vi "適應性控制_輸入權重係數+數位積分_隔振V2(實際控制).vi"() -> ()   [LabVIEW 2010]
uses:
  <vilib>/DAQmx/read.llb/DAQmx Read (Analog DBL 1Chan 1Samp).vi
  <vilib>/DAQmx/write.llb/DAQmx Write (Analog DBL 1Chan 1Samp).vi
  <vilib>/DAQmx/create/channels.llb/DAQmx Create Channel (AI-Voltage-Basic).vi
  <vilib>/DAQmx/configure/timing.llb/DAQmx Timing (Sample Clock).vi
  <vilib>/DAQmx/create/channels.llb/DAQmx Create Channel (AO-Voltage-Basic).vi
  <vilib>/daqmx/miscellaneous.llb/DAQmx Fill In Error Info.vi
  <vilib>/measure/maspectr.llb/FFT Spectrum (Mag-Phase) for 1 Chan.vi
  <vilib>/measure/NI_MAPro.lvlib
panel:
  in  "權重":dbl[][](array[numeric])=array3077x82[252314 elements]
  in  "輸出DC濾除":dbl
  out "當前權重":dbl[](array[numeric])
  in  "相位":dbl
  in  "頻率":dbl
  in  "averaging parameters":T1={"averaging mode"=enum."No averaging", "weighting mode"=enum."Exponential", "number of averages"=10} {"number of averages" min=1}
  in  "I增益":dbl
  out "magnitude":cluster{"f0":dbl, "df":dbl, "magnitude":dbl[]} {"magnitude" format="%.2p"; "f0" format="%0.2p"; "df" format="%0.2p"}
  out "Waveform Graph":cluster{"f0":dbl, "df":dbl, "magnitude":dbl[]}(graph)
  in  "DAQ input":tag
  in  "DAQ output":tag
  in  "平均數":i32=1
  in  "ÂoDC«á©ñ¤j":dbl=1.0
  in  "Kp":dbl
  out "當下誤差":dbl=0.1 format="%#_13g"
  out "模擬輸入x(t)":dbl[][](graph)
  out "理想與FIR輸出":dbl[][](graph)
  out "message":string=" INSTRUCTIONS:\r\rNormal Use:  When using subVIs that incorporate the error in/error out (or error I/O) structure, place this handler where you want to inform the user of an error, typically at the end of the I/O data path, as the last action of the program.  If the error in error? is ERROR, the handler creates a message describing the error and its source.  If the type of dialog = 1 (default), the message is displayed to the user, who can only acknowedge it.  If the type = 2, the user can acknowledge the message or abort execution; aborting a program with active I/O is not recommended.  If the type = 0, no message is displayed; this is used to process the error programmatically, and the error out cluster elements are wired to individual terminals for that reason.  \r\rOther Use:\n\r\nlocal testing.  To test the error code of a subVI or function that does not have the error I/O structure, you can wire its error code and a source string to the local error code and error source inputs.  If error in error? indicates no error and error code is not equal to 0, the local code and source are substituted for the error in values, and error? is set TRUE (ERROR)."
  out "誤差":dbl(graph)
  out "while平均運行時間":dbl
  out "收斂time":dbl
  out "各頻率誤差已達標準":bool
  in  "各頻率誤差低於多少亮燈":dbl=0.1 format="%#_13g"
  in  "order":i32=80
  in  "取樣頻率":dbl=1000.0 min=1.0 max=1000.0 step=1.0
  in  "stop":bool
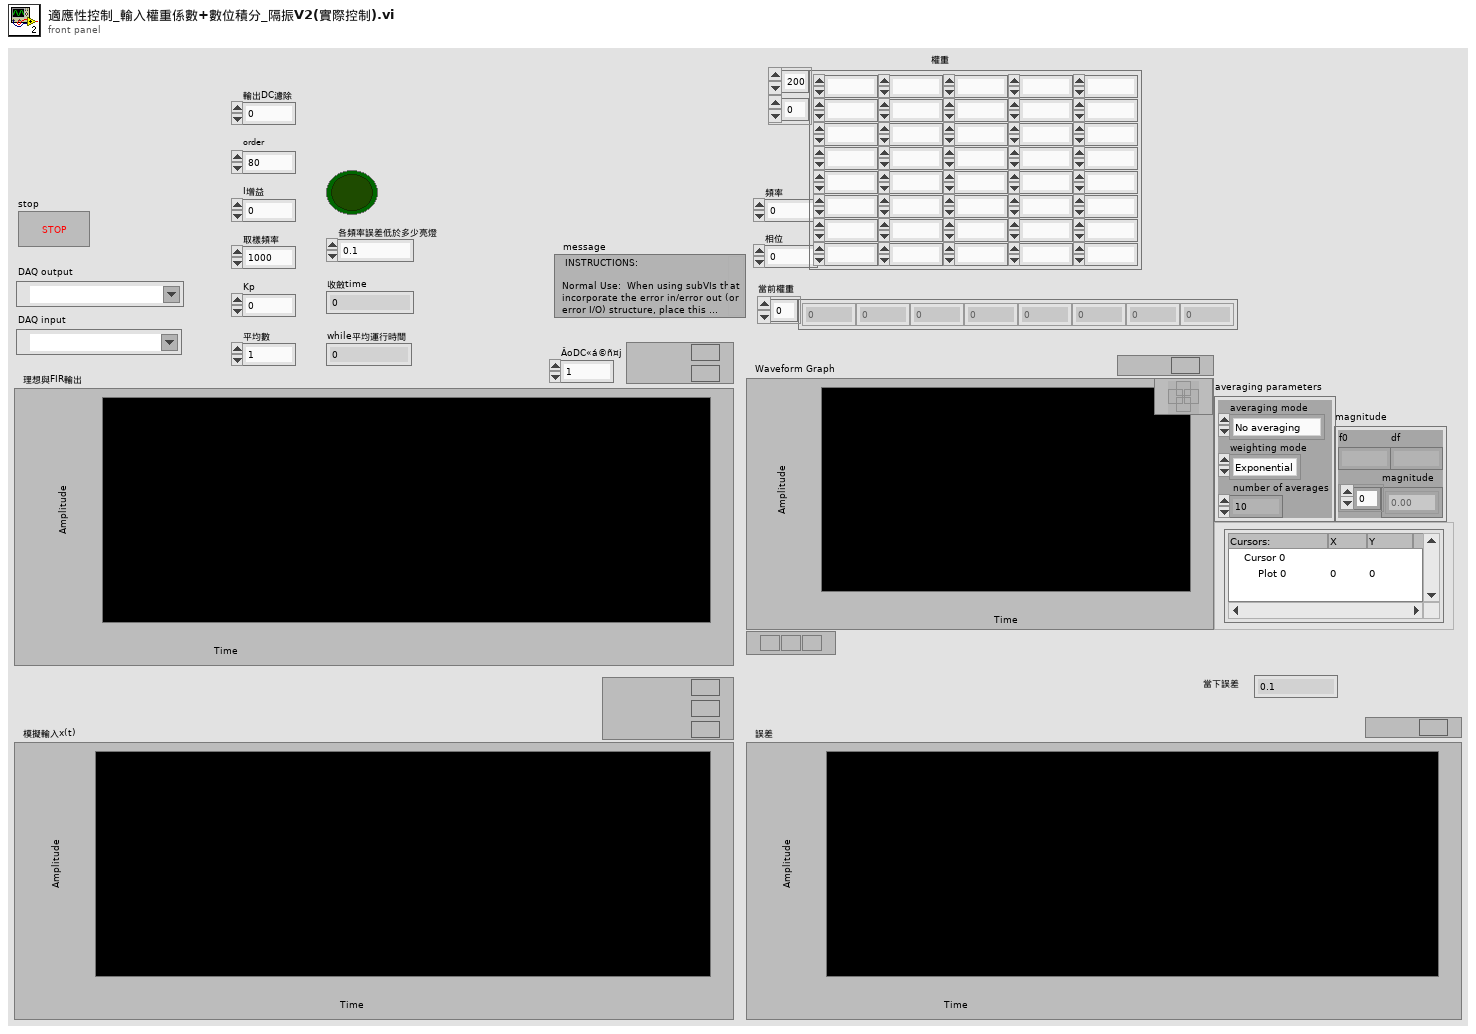
[diagram p1: front panel]
types:
  T1 = cluster{"averaging mode":enum16{"No averaging", "Vector averaging", "RMS averaging", "Peak hold"}, "weighting mode":enum16{"Linear", "Exponential"}, "number of averages":u32}
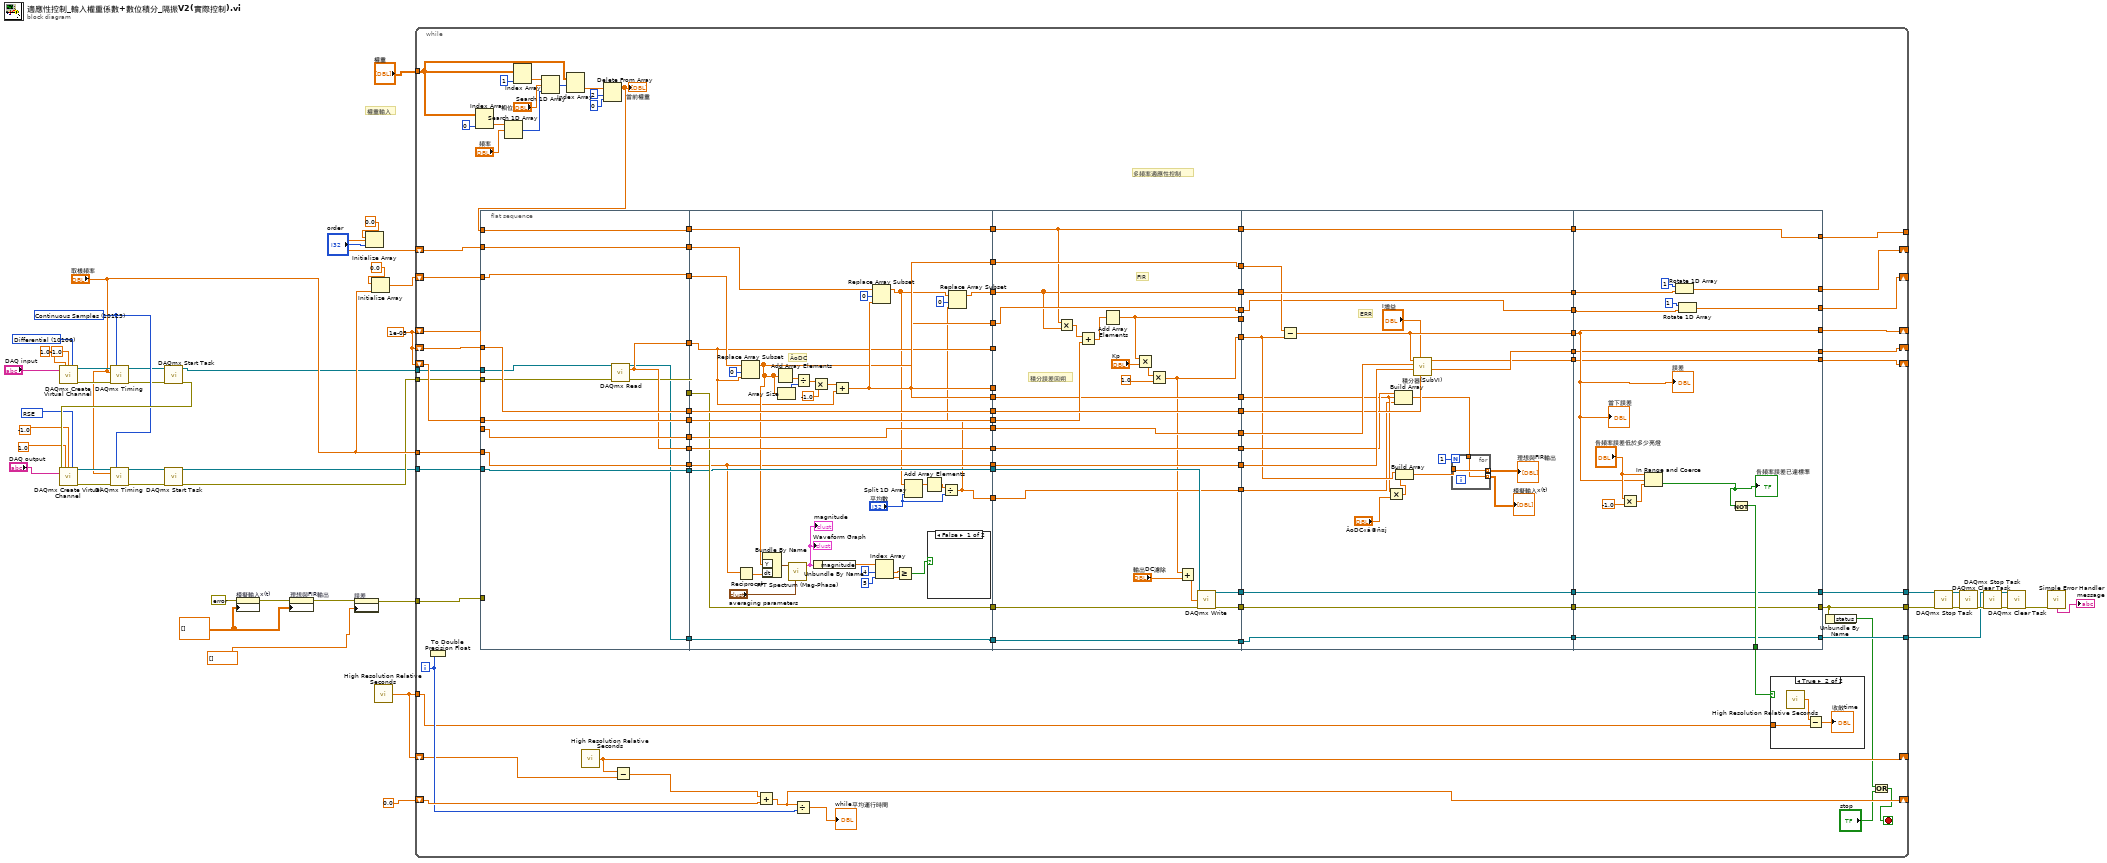
[diagram p0: block diagram]
diagram:
  w29 = 10123 items=["Finite Samples"=10178, "Continuous Samples"=10123, "Hardware Timed Single Point"=12522] ("sample mode")
  w26 = 10083 items=["Default"=-1, "RSE"=10083, "Differential"=10106, "Pseudodifferential"=12529] ("output terminal configuration")
  w25 = 10106 items=["default"=-1, "RSE"=10083, "NRSE"=10078, "Differential"=10106, "Pseudodifferential"=12529] ("input terminal configuration")
  w37 = 1e-05 ("x")
  w33 = dbl[][] [] ("History Data")
  # "權重輸入"
  n1 = call-poly <vilib>:"DAQmx Create Virtual Channel.vi"("maximum value"=1.0, "minimum value"=-1.0, "input terminal configuration"=w25, "physical channels"="DAQ input") -> ("task out"=w17:refnum<k21>, "error out"=w20:errorcluster)  [unwired: 10 in]
  n2 = call-poly <vilib>:"DAQmx Timing.vi"("task/channels in"=w17, "sample mode"=w29, "rate"="取樣頻率", "error in"=w20) -> ("task out"=w18:refnum<k21>, "error out"=w19:errorcluster)  [unwired: 10 in]
  n3 = call <vilib>:"DAQmx Start Task.vi"("task/channels in"=w18, "error in"=w19) -> ("task out"=w15:refnum<k21>, "error out"=w32:errorcluster)  [unwired: 12 in]
  n4 = call-poly <vilib>:"DAQmx Create Virtual Channel.vi"("maximum value"=1.0, "minimum value"=-1.0, "output terminal configuration"=w26, "physical channels"="DAQ output", "error in"=w32) -> ("task out"=w24:refnum<k21>, "error out"=w21:errorcluster)  [unwired: 9 in]
  n5 = call-poly <vilib>:"DAQmx Timing.vi"("task/channels in"=w24, "sample mode"=w29, "rate"="取樣頻率", "error in"=w21) -> ("task out"=w23:refnum<k21>, "error out"=w22:errorcluster)  [unwired: 10 in]
  n6 = call <vilib>:"DAQmx Start Task.vi"("task/channels in"=w23, "error in"=w22) -> ("task out"=w13:refnum<k21>, "error out"=w14:errorcluster)  [unwired: 12 in]
  n7 = property on="模擬輸入x(t)" class="WFChart (strict)"(error in=errorcluster {"status"=FALSE, "code"=0, "source"=""} ("error constant"), "History Data"=w33) -> (error out=w41:errorcluster)  [unwired: 1 in, 1 out]
  n8 = property on="理想與FIR輸出" class="WFChart (strict)"(error in=w41, "History Data"=w33) -> (error out=w42:errorcluster)  [unwired: 1 in, 1 out]
  n9 = property on="誤差" class="WFChart (strict)"(error in=w42, "History Data"=dbl[] []) -> (error out=w44:errorcluster)  [unwired: 1 in, 1 out]
  n10 = Initialize Array(0.0 ("element"), "order") -> (w36:dbl[])
  n11 = Initialize Array(0.0 ("element"), "取樣頻率") -> (w34:dbl[])
  n12 = call <vilib>:"High Resolution Relative Seconds.vi"() -> ("relative seconds"=w46:dbl)
  n13 = while {
    shift-right: [w118] -> _
    shift-left: w36 -> [w142]
    tunnel: w46 -> [w126]
    shift-right: [w127] -> _
    shift-left: w46 -> [w125]
    shift-right: [w128] -> _
    shift-left: 0.0 -> [w130]
    tunnel: w44 -> [w122]
    shift-right: [w116] -> _
    shift-left: w37 -> [w112]
    shift-right: [w108] -> _
    shift-left: w37 -> [w103]
    shift-right: [w102] -> _
    shift-left: w37 -> [w98]
    tunnel: "取樣頻率" -> [w97]
    tunnel: [w92] -> _
    shift-right: [w89] -> _
    shift-left: w34 -> [w91]
    tunnel: w15 -> [w81]
    tunnel: w14 -> [w80]
    tunnel: w13 -> [w79]
    tunnel: [w74] -> w7
    tunnel: [w64] -> w6
    tunnel: [w67] -> w5
    tunnel: "權重" -> [w49]
    i -> [w129]
    stop <- w66 stop-if-true
    # "多頻率適應性控制"
    n14 = To Double Precision Float(number=w129) -> ()  [unwired: 1 out]
    n15 = Index Array(array=w49, index (col)=0 ("disabled index (col)")) -> (element=w59:dbl[])  [unwired: 1 in]
    n16 = flat-sequence {
      tunnel: [w159] -> w143
      tunnel: w142 -> [w159]
      tunnel: [w150] -> w141
      tunnel: [w158] -> w138
      tunnel: w48 -> [w158]
      tunnel: w122 -> [_]
      tunnel: [w150] -> w119
      tunnel: [w157] -> w113
      tunnel: w112 -> [w157]
      tunnel: [w156] -> w109
      tunnel: w97 -> [w156]
      tunnel: [w155] -> w104
      tunnel: w103 -> [w155]
      tunnel: [w154] -> w99
      tunnel: w98 -> [w154]
      tunnel: [w149] -> w96
      tunnel: w91 -> [w153]
      tunnel: [w153] -> w90
      tunnel: w81 -> [w152]
      tunnel: w80 -> [w151]
      tunnel: w79 -> [w148]
      tunnel: [w148] -> w77
      tunnel: [w147] -> w70
      tunnel: w143 -> [w196]
      tunnel: w141 -> [w164]
      tunnel: [w162] -> w140
      tunnel: [w197] -> w139
      tunnel: w138 -> [w197]
      tunnel: [w190] -> w123
      tunnel: [w195] -> w120
      tunnel: w119 -> [w195]
      tunnel: [w193] -> w114
      tunnel: w113 -> [w193]
      tunnel: [w167] -> w110
      tunnel: w109 -> [w167]
      tunnel: [w192] -> w105
      tunnel: w104 -> [w192]
      tunnel: [w191] -> w100
      tunnel: w99 -> [w191]
      tunnel: w96 -> [w190]
      tunnel: [w182] -> w94
      tunnel: w90 -> [w188]
      tunnel: [w169] -> w86
      tunnel: [w182] -> w85
      tunnel: [w182] -> w83
      tunnel: [w160] -> w82
      tunnel: [w178] -> w78
      tunnel: w77 -> [w178]
      tunnel: [w177] -> w71
      tunnel: w70 -> [w177]
      tunnel: [w164] -> w61
      tunnel: w140 -> [w202]
      tunnel: w139 -> [w204]
      tunnel: [w204] -> w137
      tunnel: [w203] -> w136
      tunnel: [w202] -> w135
      tunnel: w123 -> [w209]
      tunnel: [w201] -> w121
      tunnel: w120 -> [w201]
      tunnel: [w222] -> w115
      tunnel: w114 -> [w222]
      tunnel: [w221] -> w111
      tunnel: w110 -> [w221]
      tunnel: [w220] -> w106
      tunnel: w105 -> [w220]
      tunnel: w100 -> [w218]
      tunnel: [w214] -> w95
      tunnel: w94 -> [w214]
      tunnel: [w198] -> w93
      tunnel: [w212] -> w87
      tunnel: w86 -> [w212]
      tunnel: w85 -> [w213]
      tunnel: [w213] -> w84
      tunnel: w83 -> [_]
      tunnel: w82 -> [w205]
      tunnel: w78 -> [w210]
      tunnel: [w208] -> w75
      tunnel: [w207] -> w73
      tunnel: w71 -> [w206]
      tunnel: [w206] -> w69
      tunnel: [w205] -> w62
      tunnel: w61 -> [_]
      tunnel: w137 -> [w242]
      tunnel: w136 -> [_]
      tunnel: w135 -> [w244]
      tunnel: [w244] -> w134
      tunnel: [w240] -> w133
      tunnel: w121 -> [w233]
      tunnel: [w242] -> w117
      tunnel: w115 -> [w241]
      tunnel: w111 -> [w239]
      tunnel: [w238] -> w107
      tunnel: w106 -> [w237]
      tunnel: [w236] -> w101
      tunnel: w95 -> [w235]
      tunnel: w93 -> [w231]
      tunnel: [w234] -> w88
      tunnel: w87 -> [w234]
      tunnel: w84 -> [w230]
      tunnel: [w227] -> w76
      tunnel: w75 -> [w227]
      tunnel: w73 -> [w226]
      tunnel: [w226] -> w72
      tunnel: w69 -> [w225]
      tunnel: [w225] -> w68
      tunnel: w62 -> [w224]
      tunnel: w134 -> [w261]
      tunnel: [w267] -> w118
      tunnel: w133 -> [w258]
      tunnel: [w263] -> w124
      tunnel: [w259] -> w92
      tunnel: w117 -> [w259]
      tunnel: [w258] -> w116
      tunnel: [w257] -> w108
      tunnel: w107 -> [w257]
      tunnel: [w256] -> w102
      tunnel: w101 -> [w256]
      tunnel: [w254] -> w89
      tunnel: w88 -> [w253]
      tunnel: w76 -> [w252]
      tunnel: [w252] -> w74
      tunnel: [w251] -> w64
      tunnel: w72 -> [w251]
      tunnel: w68 -> [w250]
      tunnel: [w250] -> w67
      frame #0 {
        n17 = call-poly <vilib>:"DAQmx Read.vi"("task/channels in"=w152, "error in"=w151) -> ("task out"=w147:refnum<k21>, "data"=w150:dbl, "error out"=w149:errorcluster)  [unwired: 11 in]
      }
      frame #1 {
        # "ÂoDC"
        n18 = Reciprocal(x=w167) -> (1/x=w166:dbl)
        n19 = Replace Array Subset(array=w188, new element=w164, index=0) -> (w169:dbl[])
        n20 = Bundle By Name("Y"=w169, "dt"=w166) -> (w176:waveform(dbl))  [unwired: 1 in]
        n21 = Add Array Elements(numeric array=w169) -> (sum=w187:dbl)
        n22 = Array Size(array=w169) -> (size(s)=w186:i32)
        n23 = call-poly <vilib>:"FFT Spectrum (Mag-Phase).vi"("averaging parameters"="averaging parameters", "time signal"=w176) -> ("magnitude"=w175:cluster{"f0":dbl, "df":dbl, "magnitude":dbl[]})  [unwired: 5 in, 4 out]
        "Waveform Graph" <- w175
        "magnitude" <- w175
        n24 = Divide(x=w187, y=w186) -> (x/y=w185:dbl)
        n25 = Multiply(x=w185, y=-1.0) -> (x*y=w183:dbl)
        n26 = Unbundle By Name(w175) -> ("magnitude"=w174:dbl[])
        n27 = Add(x=w183, y=w164) -> (x+y=w182:dbl)
        n28 = Replace Array Subset(array=w196, new element=w182, index=0) -> (w163:dbl[])
        n29 = Index Array(array=w174, index #1=4 ("index"), index #2=5 ("index")) -> (element #1=w171:dbl, element #2=w170:dbl)
        n30 = Greater Or Equal?(x=w171, y=w170) -> (x >= y?=w168:bool)
        n31 = Split 1D Array(array=w163, index="平均數") -> (first subarray=w181:dbl[])  [unwired: 1 out]
        n32 = Add Array Elements(numeric array=w181) -> (sum=w180:dbl)
        n33 = case shown="False" w168 {
          frame False {
          }
          frame True {
          }
        }
        n34 = Divide(x=w180, y="平均數") -> (x/y=w160:dbl)
        n35 = Replace Array Subset(array=w163, new element=w160, index=0) -> (w162:dbl[])
      }
      frame #2 {
        # "積分誤差回朔"
        # "FIR"
        n36 = Multiply(x=w204, y=w202) -> (x*y=w219:dbl[])
        n37 = Add(x=w219, y=w218) -> (x+y=w217:dbl[])
        n38 = Add Array Elements(numeric array=w217) -> (sum=w203:dbl)
        n39 = Multiply(x=w203, y="Kp") -> (x*y=w215:dbl)
        n40 = Multiply(x=w215, y=1.0) -> (x*y=w198:dbl)
        n41 = Add(x=w198, y="輸出DC濾除") -> (x+y=w200:dbl)
        n42 = call-poly <vilib>:"DAQmx Write.vi"("task/channels in"=w210, "data"=w200, "error in"=w209) -> ("task out"=w208:refnum<k21>, "error out"=w207:errorcluster)  [unwired: 10 in, 1 out]
      }
      frame #3 {
        # "ERR"
        n43 = Subtract(x=w235, y=w231) -> (x-y=w240:dbl)
        n44 = Multiply(x=w230, y="ÂoDC«á©ñ¤j") -> (x*y=w228:dbl)
        n45 = Build Array(w233, w230, w224) -> (w232:dbl[])
        n46 = Build Array(w231, w228) -> (w246:dbl[])
        n47 = call "積分器(SubVI).vi"("輸入累加ERR回朔"=w237, "I增益"="I增益", "samples (Hz)"=w239, "前一個ERR"=w241, "當下ERR"=w240) -> ("輸出累加ERR回朔"=w238:dbl, "積分修正量"=w236:dbl)  [unwired: 5 in]
        n48 = for {
          N: 1 -> [_]
          tunnel: [w249] -> w243 mode=indexing
          tunnel: w246 -> [w249]
          tunnel: [w248] -> w245 mode=indexing
          tunnel: w232 -> [w248]
        }
        "理想與FIR輸出" <- w243
        "模擬輸入x(t)" <- w245
      }
      frame #4 {
        n49 = Multiply(x="各頻率誤差低於多少亮燈", y=-1.0) -> (x*y=w264:dbl)
        n50 = In Range and Coerce(upper limit="各頻率誤差低於多少亮燈", x=w258, lower limit=w264) -> (In Range?=w260:bool)  [unwired: 1 out]
        "各頻率誤差已達標準" <- w260
        n51 = Rotate 1D Array(1:w261, 2:1 ("n")) -> (0:w267:dbl[])
        n52 = Rotate 1D Array(1:w253, 2:1 ("n")) -> (0:w254:dbl[])
        n53 = Not(x=w260) -> (.not. x?=w263:bool)
        "誤差" <- w258
        "當下誤差" <- w258
      }
    }
    n54 = Search 1D Array(1D array=w59, element="頻率") -> (index of element=w56:i32)  [unwired: 1 in]
    n55 = Index Array(array=w49, index (col)=1 ("disabled index (col)")) -> (element=w57:dbl[])  [unwired: 1 in]
    n56 = Search 1D Array(1D array=w57, element="相位", start index (0)=w56) -> (index of element=w53:i32)
    n57 = Index Array(array=w49, index (row)=w53) -> (element=w52:dbl[])  [unwired: 1 in]
    n58 = call <vilib>:"High Resolution Relative Seconds.vi"() -> ("relative seconds"=w127:dbl)
    n59 = Delete From Array(array=w52, length=2, index=0) -> (array with subset deleted=w48:dbl[])  [unwired: 1 out]
    "當前權重" <- w48
    n60 = Subtract(x=w127, y=w125) -> (x-y=w132:dbl)
    n61 = Add(x=w132, y=w130) -> (x+y=w128:dbl)
    n62 = Divide(x=w128, y=w129) -> (x/y=→"while平均運行時間":dbl)
    n63 = case shown="True" w124 {
      tunnel: w126 -> [_ w144]
      frame False {
      }
      frame True {
        n64 = call <vilib>:"High Resolution Relative Seconds.vi"() -> ("relative seconds"=w146:dbl)
        n65 = Subtract(x=w146, y=w144) -> (x-y=→"收斂time":dbl)
      }
    }
    n66 = Unbundle By Name(w64) -> ("status"=w63:bool)
    n67 = Or(x=w63, y="stop") -> (x .or. y?=w66:bool)
  }
  n68 = call <vilib>:"DAQmx Stop Task.vi"("task/channels in"=w7, "error in"=w6) -> ("task out"=w8:refnum<k21>, "error out"=w9:errorcluster)  [unwired: 12 in]
  n69 = call <vilib>:"DAQmx Clear Task.vi"("task in"=w8, "error in"=w9) -> ("error out"=w12:errorcluster)  [unwired: 13 in]
  n70 = call <vilib>:"DAQmx Stop Task.vi"("task/channels in"=w5, "error in"=w12) -> ("task out"=w11:refnum<k21>, "error out"=w10:errorcluster)  [unwired: 12 in]
  n71 = call <vilib>:"DAQmx Clear Task.vi"("task in"=w11, "error in"=w10) -> ("error out"=w4:errorcluster)  [unwired: 13 in]
  n72 = call <vilib>:"Simple Error Handler.vi"("error in (no error)"=w4) -> ("message"=→"message":string)  [unwired: 4 in, 4 out]
